vi "Configure Signal.vi"(0 "Register Bus":T1, 1 "scope":string(combo)="rx", 5 "sample rate [S/s]":dbl=10000000.0 caption="Sample Rate [S/s]" min=1.0 max=250000000.0 format="%#.3pS/s", 7 "frequency [Hz]":dbl=2450000000.0 caption="Frequency [Hz]" format="%#.3pHz", 9 "level [dBm]":dbl=-10.0 caption="Level [dBm]" format="%#_gdBm", 11 "error in":errorcluster, 12 "LO source":string(combo)="LO1" caption="LO Source", 13 "LO frequency [Hz]":dbl=-1.0 caption="LO Frequency [Hz]" format="%#.3pHz") -> (3 "coerced vertical range [Vpp]":dbl caption="Coerced Vertical Range [Vpp]" format="%#.3pV", 4 "Register Bus (out)":T1, 6 "coerced sample rate [S/s]":dbl=10000000.0 caption="Coerced Sample Rate [S/s]" min=1.0 max=250000000.0 format="%#.3pS/s", 8 "coerced frequency [Hz]":dbl=2450000000.0 caption="Coerced Frequency [Hz]" format="%#.3pHz", 10 "coerced level [dBm]":dbl=-10.0 caption="Coerced Level [dBm]" format="%#_gdBm", 14 "coerced LO frequency [Hz]":dbl=-1.0 caption="coerced LO Frequency [Hz]" format="%#.3pHz", 15 "error out":errorcluster)   [LabVIEW 2017]
doc: "Configure the DSP and signal path for the device."
uses:
  <instrlib>/_niInstr/Register Bus/v0/Host/Public/Register Bus Session.ctl
  <instrlib>/_niInstr/Register Bus/v0/Host/Private/Session Data.ctl
  Rx FPGA VI Reference.ctl
  Tx FPGA VI Reference.ctl
  <vilib>/Utility/error.llb/Error Cluster From Error Code.vi
  <vilib>/rvi/errors/niLvFpgaAdjustHostInterfaceError.vi
  <vilib>/rvi/interface/nirviReadWriteControl/nirviReadWriteControl.xnode
  <instrlib>/ni579x/Config/v2/Host/ni579x Config v2 Host.lvlib
  NiFpgaLv.dll
  <vilib>/rvi/interface/Simulation/niFpgaSimulationCallBeginRW.vi
  <instrlib>/_niInstr/Register Bus/v0/Host/niInstr Register Bus v0 Host.lvlib
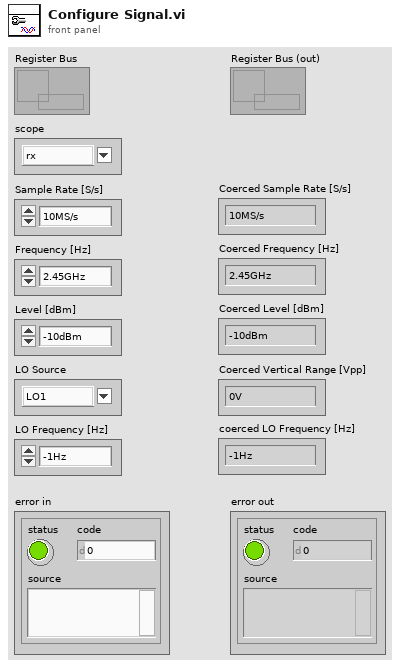
[diagram p1: front panel]
types:
  T1 = typedef "niInstr Register Bus v0 Host.lvlib/Register Bus Session.ctl" = refnum<queue>
  T2 = typedef "ni579x Config v2 Shared.lvlib/ni579x Characterization Data.ctl" = cluster{"Attenuation Table [dB]":dbl[][], "Frequencies [Hz]":dbl[], "IQ Imbalance Table":T3[], "Gain Table":T4[][]}
  T3 = typedef "ni579x Config v2 Shared.lvlib/ni579x IQ Imbalance.ctl" = cluster{"Gain Imbalance [linear]":dbl, "Phase Imbalance [radians]":dbl, "Offset":cdb}
  T4 = typedef "ni579x Config v2 Shared.lvlib/ni579x Gain to Attenuation Mapping.ctl" = cluster{"Actual Gain [dB]":dbl, "Attenuation Table Index":i32}
  T5 = typedef "niInstr DSP v1 Shared.lvlib/IQ Gain.ctl" = cluster{"gain I":fxp<+/-,24,3>, "gain Q":fxp<+/-,24,3>}
  T6 = typedef "niInstr DSP v1 Shared.lvlib/IQ Impairments.ctl" = cluster{"inline gain I":fxp<+/-,18,1>, "inline gain Q":fxp<+/-,18,1>, "cross gain I":fxp<+/-,18,1>, "cross gain Q":fxp<+/-,18,1>, "pre-gain offset I":fxp<+/-,18,1>, "pre-gain offset Q":fxp<+/-,18,1>, "post-gain offset I":fxp<+/-,18,1>, "post-gain offset Q":fxp<+/-,18,1>}
  T7 = typedef "Rx FPGA VI Reference.ctl" = refnum<k20>
  T8 = typedef "Tx FPGA VI Reference.ctl" = refnum<k20>
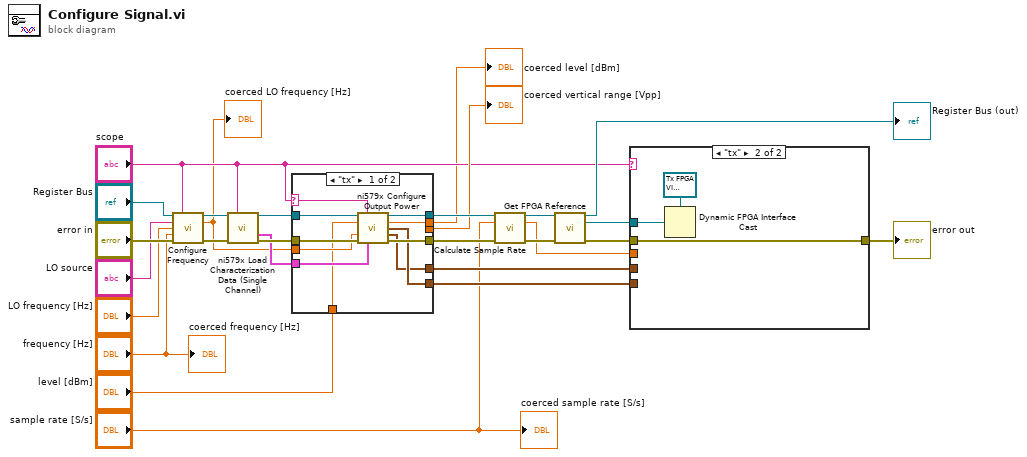
[diagram p0: block diagram]
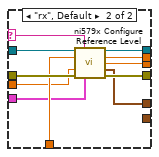
[diagram p2: hidden frame]
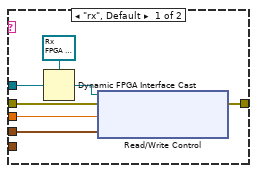
[diagram p3: hidden frame]
diagram:
  n1 = call "Configure Frequency.vi"("Register Bus"="Register Bus", "scope"="scope", "LO source"="LO source", "LO frequency [Hz]"="LO frequency [Hz]", "frequency [Hz]"="frequency [Hz]", "error in"="error in") -> ("Register Bus (out)"=w9:T1, "coerced LO frequency [Hz]"=w1:dbl, "error out"=w11:errorcluster)  [unwired: 7 in]
  "coerced LO frequency [Hz]" <- w1
  n2 = call <instrlib>:"ni579x Load Characterization Data (Single Channel).vi"("Register Bus"=w9, "scope"="scope", "Error In"=w11) -> ("Register Bus (out)"=w20:T1, "Characterization Data"=w13:T2, "Error Out"=w26:errorcluster)  [unwired: 7 in, 3 out]
  n3 = case shown="\"tx\"" "scope" {
    selector: "scope" -> [w32 w40]
    tunnel: w26 -> [w38 w49]
    tunnel: "level [dBm]" -> [w31 w48]
    tunnel: w20 -> [w34 w47]
    tunnel: [w37 w46] -> w18
    tunnel: [w33 w45] -> w17
    tunnel: [_ w44] -> w15
    tunnel: [w29 w43] -> w14
    tunnel: w13 -> [w36 w42]
    tunnel: w1 -> [w35 w41]
    tunnel: [w30 _] -> w5
    tunnel: [w28 w39] -> w4
    frame "tx" {
      n4 = call <instrlib>:"ni579x Configure Output Power.vi"("Register Bus"=w34, "scope"=w32, "output power [dBm]"=w31, "frequency [Hz]"=w35, "Error In"=w38, "characterization data"=w36) -> ("Register Bus (out)"=w33:T1, "coerced output power [dBm]"=w28:dbl, "digital gain"=w30:T5, "IQ impairment correction"=w29:T6, "Error Out"=w37:errorcluster)  [unwired: 5 in]
    }
    frame "rx", Default {
      n5 = call <instrlib>:"ni579x Configure Reference Level.vi"("Register Bus"=w47, "scope"=w40, "reference level [dBm]"=w48, "frequency [Hz]"=w41, "Error In"=w49, "characterization data"=w42) -> ("Register Bus (out)"=w45:T1, "coerced reference level [dBm]"=w39:dbl, "coerced vertical range [Vpp]"=w44:dbl, "IQ impairment correction"=w43:T6, "Error Out"=w46:errorcluster)  [unwired: 5 in]
    }
  }
  "coerced vertical range [Vpp]" <- w15
  "coerced level [dBm]" <- w4
  n6 = call "Calculate Sample Rate.vi"("Register Bus"=w17, "sample rate [S/s]"="sample rate [S/s]", "error in"=w18) -> ("Register Bus (out)"=w19:T1, "sample rate [ratio]"=w25:dbl, "error out"=w27:errorcluster)  [unwired: 10 in]
  n7 = call <instrlib>:"Get FPGA Reference.vi"("session in"=w19, "error in"=w27) -> ("session out"=→"Register Bus (out)":T1, "fpga ref"=w24:refnum<k20>, "error out"=w22:errorcluster)  [unwired: 11 in]
  n8 = case shown="\"tx\"" "scope" {
    tunnel: w25 -> [w56 _]
    tunnel: w24 -> [w55 w59]
    tunnel: [w54 w57] -> w23
    tunnel: w22 -> [w53 w57]
    tunnel: w14 -> [w50 _]
    tunnel: w5 -> [_ _]
    frame "rx", Default {
      n9 = Dynamic FPGA Interface Cast(Session In=T7 refnum ("FPGA VI Reference Out"), Type=w55) -> (Session Out=w51:T7)
      n10 = xnode "Read/Write Control"("FPGA VI Reference In"=w51, "error in"=w53, "rx.output sample rate"=w56, "rx.impairments"=w50) -> ("error out"=w54:errorcluster)  [unwired: 1 out]
    }
    frame "tx" {
      n11 = Dynamic FPGA Interface Cast(Session In=T8 refnum ("FPGA VI Reference Out"), Type=w59) -> ()  [unwired: 1 out]
    }
  }
  "error out" <- w23
  "coerced sample rate [S/s]" <- "sample rate [S/s]"
  "coerced frequency [Hz]" <- "frequency [Hz]"
